vi "Get Device Parameters.vi"(8 "error in":errorcluster, 11 "Ballard ARINC 429 custom device in":T3=18446744073709551615 format="%.0x") -> (0 "error out":errorcluster, 2 "device parameters":T1, 3 "Ballard ARINC 429 custom device out":T3 format="%.0x")   [LabVIEW 2020, in "Ballard ARINC 429 Scripting.lvlib"]
doc: "Returns hardware device parameters such as <b>PXI slot number</b> and <b>core number</b>."
uses:
  Ballard ARINC 429 Scripting.lvlib
  <vilib>/NI VeriStand/Custom Device API/Custom Device Item Ref.ctl
  Shared/Device Parameters.ctl
  Shared/Initialization Method.ctl
  Constants.vi
  <vilib>/NI VeriStand/Custom Device API/Get Item Property (U16).vi
  <vilib>/NI VeriStand/Custom Device API/Get Item Property (I32).vi
  <vilib>/NI VeriStand/Custom Device API/Custom Device API.lvlib
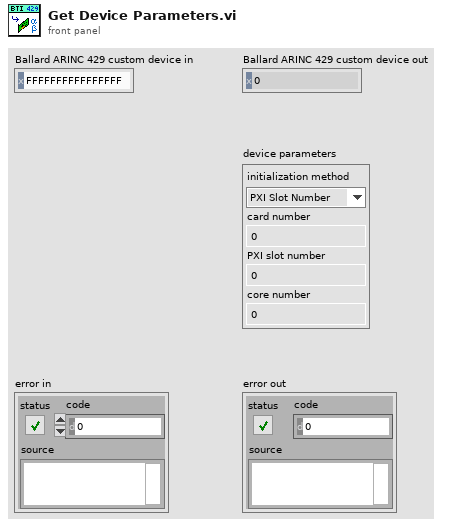
[diagram p1: front panel]
types:
  T1 = typedef "Device Parameters.ctl" = cluster{"initialization method":T2, "card number":i32, "PXI slot number":i32, "core number":i32}
  T2 = typedef "Initialization Method.ctl" = enum16{"PXI Slot Number", "Card Number"}
  T3 = typedef "Custom Device API.lvlib/Custom Device Item Ref.ctl" = u64
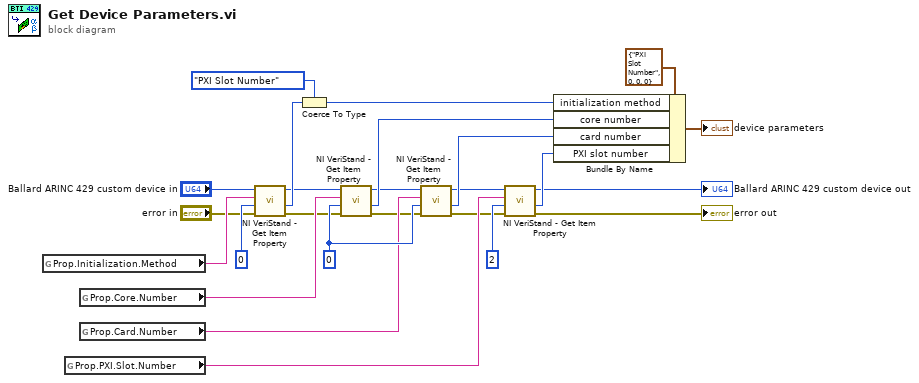
[diagram p0: block diagram]
diagram:
  w23 = 0 ("Default Value")
  n1 = global read "Constants.vi" "Prop.Initialization.Method"() -> (w18:string)
  n2 = global read "Constants.vi" "Prop.PXI.Slot.Number"() -> (w19:string)
  n3 = global read "Constants.vi" "Prop.Core.Number"() -> (w21:string)
  n4 = global read "Constants.vi" "Prop.Card.Number"() -> (w20:string)
  n5 = call-poly <vilib>:"NI VeriStand - Get Item Property.vi"("error in (no error)"="error in", "Default Value"=u16 0, "Property Name"=w18, "Item Ref in"="Ballard ARINC 429 custom device in") -> ("error out"=w5:errorcluster, "Value"=w14:u16, "Item Ref out"=w4:T3)  [unwired: 4 in, 1 out]
  n6 = Coerce To Type(0:w14, 1:Initialization_Method."PXI Slot Number" ("initialization method")) -> (2:w3:T2)
  n7 = call-poly <vilib>:"NI VeriStand - Get Item Property.vi"("error in (no error)"=w5, "Default Value"=w23, "Property Name"=w21, "Item Ref in"=w4) -> ("error out"=w11:errorcluster, "Value"=w17:i32, "Item Ref out"=w12:T3)  [unwired: 4 in, 1 out]
  n8 = call-poly <vilib>:"NI VeriStand - Get Item Property.vi"("error in (no error)"=w11, "Default Value"=w23, "Property Name"=w20, "Item Ref in"=w12) -> ("error out"=w9:errorcluster, "Value"=w16:i32, "Item Ref out"=w10:T3)  [unwired: 4 in, 1 out]
  n9 = call-poly <vilib>:"NI VeriStand - Get Item Property.vi"("error in (no error)"=w9, "Default Value"=2, "Property Name"=w19, "Item Ref in"=w10) -> ("error out"=→"error out":errorcluster, "Value"=w15:i32, "Item Ref out"=→"Ballard ARINC 429 custom device out":T3)  [unwired: 4 in, 1 out]
  n10 = Bundle By Name(cluster=T1 {"initialization method"=enum."PXI Slot Number", "card number"=0, "PXI slot number"=0, "core number"=0} ("device parameters"), "initialization method"=w3, "core number"=w17, "card number"=w16, "PXI slot number"=w15) -> (→"device parameters":T1)
